vi "Gripper Controller.vi"(8 "error in":errorcluster) -> ()   [LabVIEW 2017]
doc: "This VI executes continuously carrying out the current operation and responding to updates or new operations. It will often contain the timing or control code that is difficult to place directly in TeleOp. This VI generally opens all sensors and motors and isolates the rest of the robot code from knowing how the operations are carried out."
uses:
  <vilib>/Rock Robotics/WPI/Framework/Completion Status.ctl
  Gripper Setpoints.ctl
  Gripper Operations.ctl
  <vilib>/Rock Robotics/SystemInterfaces/DIO/FPGA_DIOPWMChannel.ctl
  <vilib>/Rock Robotics/Network Tables/NT Write Boolean.vi
panel:
  in  "Interactive Values":T1
  out "Current\nCmd":string
  in  "Buttons":cluster{"Execute Cmd":bool, "Abort Cmd":bool}
  out "Command Timing":cluster{"Start Time (ms)":u32, "Iterations":i32}
  out "Status":T3
  # "Tip: It may be helpful to observe inputs and sensor values.\nYou may also want to display tuning or debugging controls."
  # "Interactive Command: You may fill in the settings for a command\nand schedule it with the Execute button. You can observe and abort\nany command while fine tuning the code for the controller."
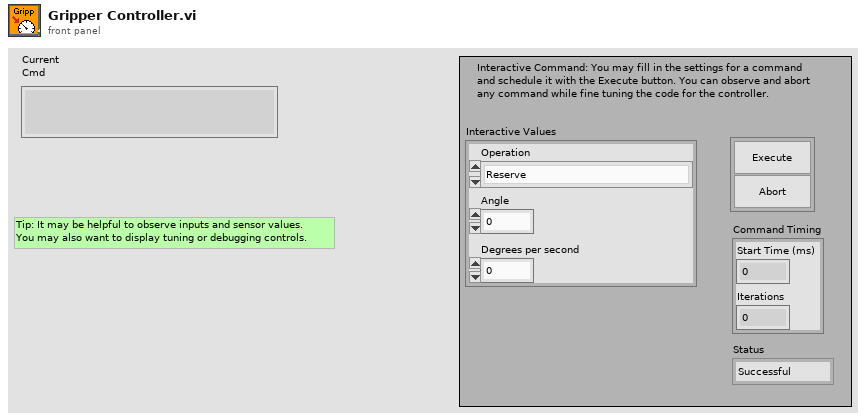
[diagram p1: front panel]
types:
  T1 = typedef "Gripper Setpoints.ctl" = cluster{"Operation":T2, "Angle":dbl, "Degrees per second":dbl}
  T2 = typedef "Gripper Operations.ctl" = enum16{"Reserve", "Read Current", "Immediate", "Grip Power Cube", "Release Power Cube"}
  T3 = typedef "Completion Status.ctl" = enum16{"Successful", "Aborted", "Incomplete"}
  T4 = typedef "FPGA_DIOPWMChannel.ctl" = enum8{"PWM 0", "PWM 1", "PWM 2", "PWM 3", "PWM 4", "PWM 5", "PWM 6", "PWM 7", "PWM 8", "PWM 9", "PWM MXP 0", "PWM MXP 1", "PWM MXP 2", "PWM MXP 3", "PWM MXP 4", "PWM MXP 5", "PWM MXP 6", "PWM MXP 7", "PWM MXP 8", "PWM MXP 9", "Invalid"}
  T5 = typedef "WPI_ServoDeviceRef.ctl" = cluster{"DeviceStatus":errorcluster, "PWM Channel":T4, "DeadBand":T6}
  T6 = typedef "WPI_PWMDeadband.ctl" = cluster{"Name":string, "maxPositivePwm":i32, "minPositivePwm":i32, "centerPwm":i32, "maxNegativePwm":i32, "minNegativePwm":i32, "angularRange":u16}
  T7 = typedef "Command Status Info.ctl" = cluster{"Name":string, "Status":T3, "notifier out":T8}
  T8 = typedef "Completion Notifier.ctl" = refnum<notifier>
  T9 = cluster{"Current Command":T1, "Command Timing":cluster{"Start Time (ms)":u32, "Iterations":i32}, "Command Arguments":cluster{"Command Info":T7, "Description":string, "Default Command":T1, "queue out":refnum<queue>, "Subsystem Name":string}}
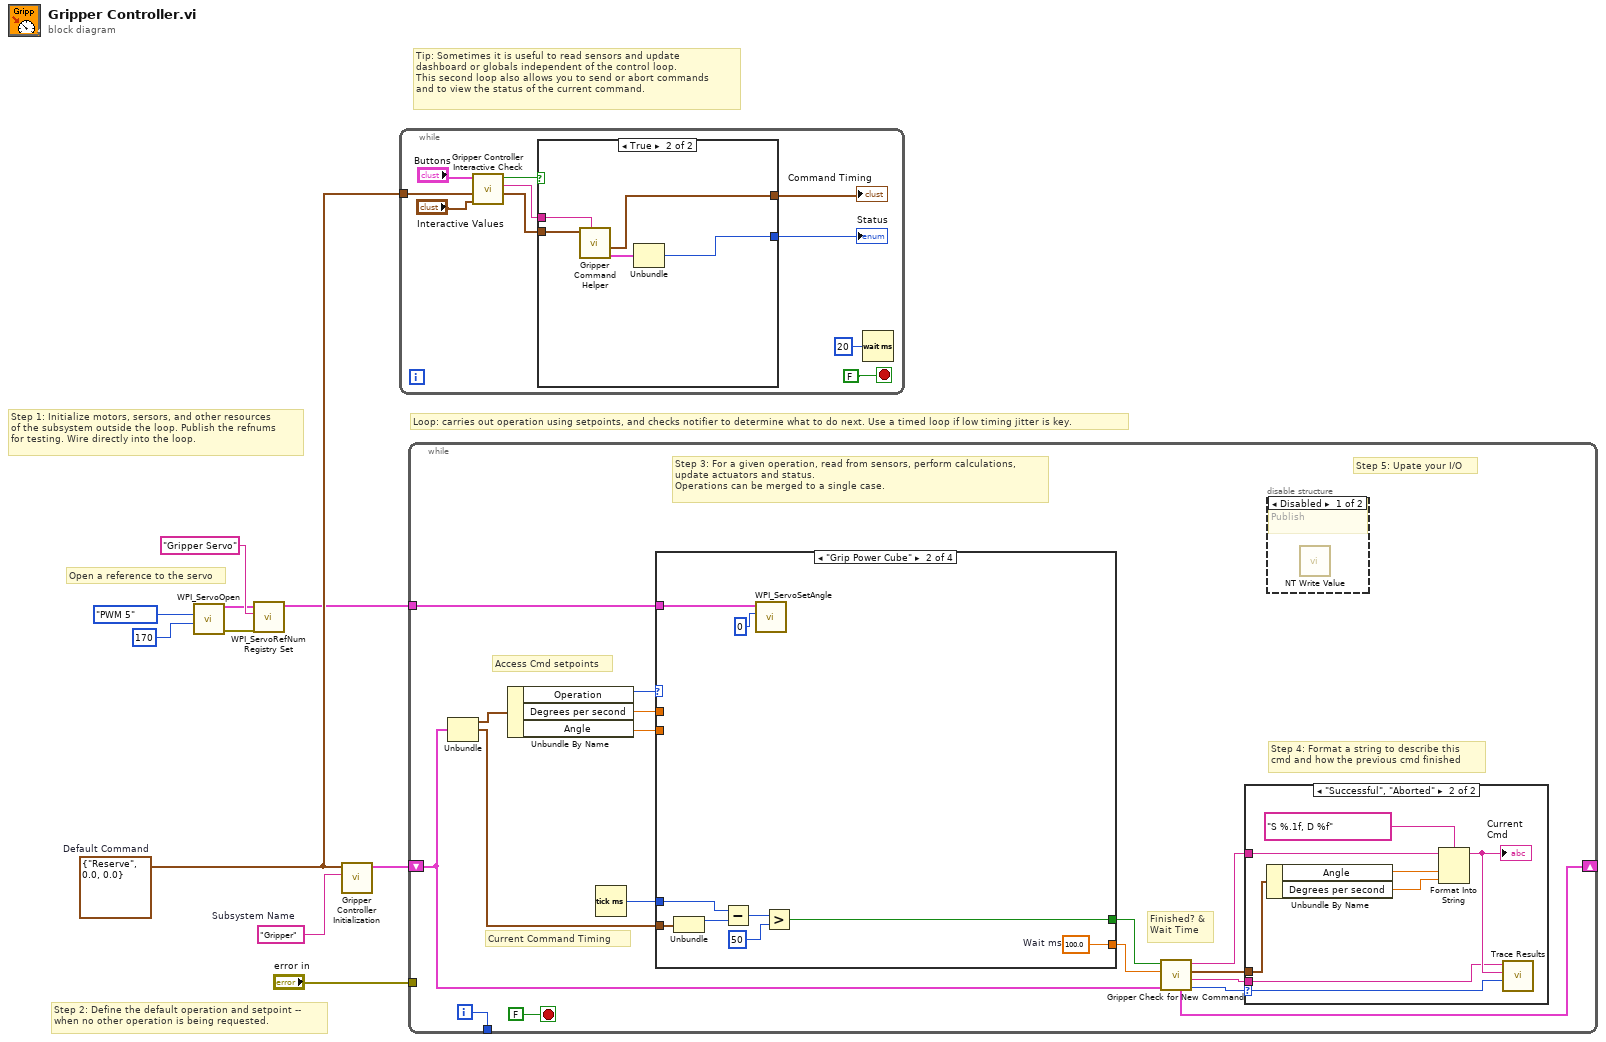
[diagram p0: block diagram]
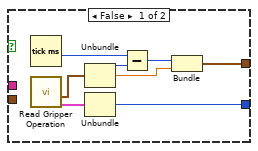
[diagram p2: hidden frame]
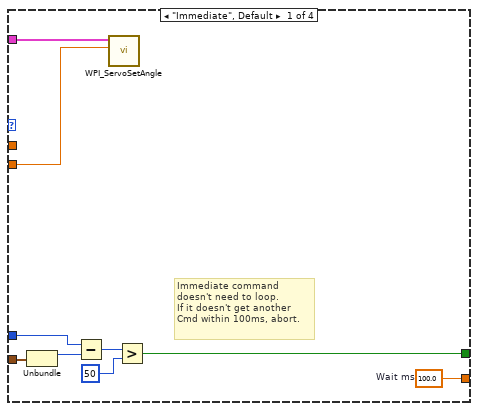
[diagram p5: hidden frame]
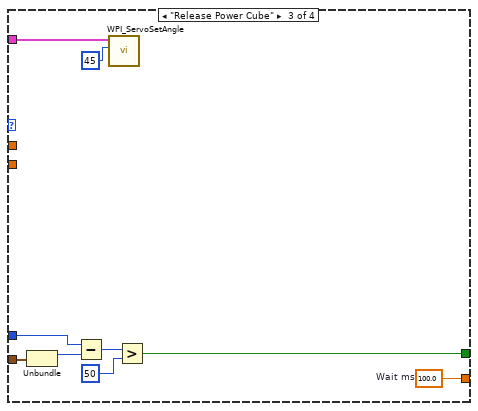
[diagram p6: hidden frame]
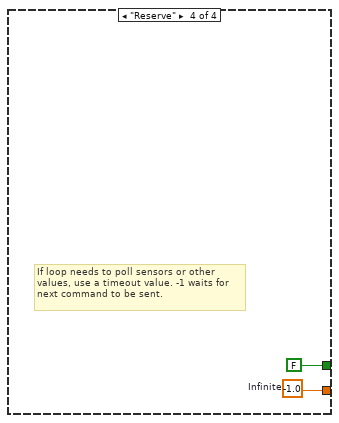
[diagram p7: hidden frame]
diagram:
  w7 = T1 {"Operation"=enum."Reserve", "Angle"=0.0, "Degrees per second"=0.0}  # Default Command
  w8 = "Gripper"  # Subsystem Name
  # "Open a reference to the servo"
  # "Tip: Sometimes it is useful to read sensors and update\ndashboard or globals independent of the control loop.\nThis second loop also allows you to send or abort commands\nand to view the status of the current command."
  # "Step 2: Define the default operation and setpoint --\nwhen no other operation is being requested."
  # "Step 1: Initialize motors, sersors, and other resources\nof the subsystem outside the loop. Publish the refnums\nfor testing. Wire directly into the loop."
  # "Loop: carries out operation using setpoints, and checks notifier to determine what to do next. Use a timed loop if low timing jitter is key."
  n1 = call <vilib>:"WPI_ServoOpen.vi"("Angular Range"=u16 170, "PWM Channel"=FPGA_DIOPWMChannel."PWM 5") -> ("error out"=w4:errorcluster, "ServoDeviceRef"=w5:T5)  [unwired: 2 in, 6 out]
  n2 = call <vilib>:"WPI_ServoRefNum Registry Set.vi"("error in (no error)"=w4, "refnum name"="Gripper Servo", "ServoDeviceRef"=w5) -> ("ServoDeviceRef"=w1:T5)  [unwired: 7 in, 1 out]
  n3 = call "Gripper Controller Initialization.vi"("Subsystem Name"=w8, "Default Command"=w7) -> ("Current Command"=w9:T9)  [unwired: 9 in]
  n4 = while {
    tunnel: w7 -> [w17]
    stop <- FALSE stop-if-true
    n5 = call "Gripper Controller Interactive Check.vi"("Interactive Command in"="Interactive Values", "Default Command"=w17, "Buttons"="Buttons") -> ("Interactive Command out"=w14:T1, "Trace String"=w15:string, "Schedule"=w16:bool)  [unwired: 6 in]
    n6 = case shown="True" w16 {
      tunnel: [w28 w33] -> w13
      tunnel: w14 -> [_ w31]
      tunnel: [w24 w29] -> w12
      tunnel: w15 -> [_ w32]
      frame False {
        n7 = Tick Count (ms)() -> (millisecond timer value=w23:u32)
        n8 = call "Read Gripper Operation.vi"() -> ("Command Info"=w21:T7, "SubSystem Data"=w22:T1)  [unwired: 9 in, 1 out]
        n9 = Unbundle(w22) -> ("Operation"=w27:T2, "Angle"=w25:dbl)  [unwired: 1 out]
        n10 = Unbundle(w21) -> ("Status"=w28:T3)  [unwired: 2 out]
        n11 = Subtract(x=w23, y=w27) -> (x-y=w26:u32)
        n12 = Bundle(w26, "Angle"=w25) -> (w24:cluster{u32, "Angle":dbl})  [unwired: 1 in]
      }
      frame True {
        n13 = call "Gripper Command Helper.vi"("Description"=w32, "SubSystem Data"=w31) -> ("Command Info Out"=w30:T7, "Command Timing"=w29:cluster{"Start Time (ms)":u32, "Iterations":i32})  [unwired: 7 in, 1 out]
        n14 = Unbundle(w30) -> ("Status"=w33:T3)  [unwired: 2 out]
      }
    }
    "Status" <- w13
    "Command Timing" <- w12
    n15 = Wait (ms)(milliseconds to wait=u32 20) -> ()  [unwired: 1 out]
  }
  n16 = while {
    shift-right: [w42] -> _
    shift-left: w9 -> [w35]
    tunnel: [w49] -> _
    tunnel: "error in" -> [_]
    tunnel: w1 -> [w34]
    i -> [w49]
    stop <- FALSE stop-if-true
    # "Step 5: Upate your I/O"
    # "Step 4: Format a string to describe this\ncmd and how the previous cmd finished"
    # "Current Command Timing"
    # "Access Cmd setpoints"
    # "Finished? &\nWait Time"
    # "Step 3: For a given operation, read from sensors, perform calculations,\nupdate actuators and status.\nOperations can be merged to a single case."
    n17 = Unbundle(w35) -> ("Current Command"=w48:T1, "Command Timing"=w44:cluster{"Start Time (ms)":u32, "Iterations":i32})  [unwired: 1 out]
    n18 = Unbundle By Name(w48) -> ("Operation"=w47:T2, "Degrees per second"=w46:dbl, "Angle"=w43:dbl)
    n19 = Tick Count (ms)() -> (millisecond timer value=w45:u32)
    n20 = case shown="\"Grip Power Cube\"" w47 {
      tunnel: [w67 w76 w85 w87] -> w40
      tunnel: [w61 w70 w79 FALSE ("ignore previous (F)")] -> w41
      tunnel: w44 -> [w63 w72 w81 _]
      tunnel: w46 -> [_ _ _ _]
      tunnel: w45 -> [w62 w71 w80 _]
      tunnel: w43 -> [w59 _ _ _]
      tunnel: w34 -> [w60 w68 w77 _]
      frame "Immediate", Default {
        w67 = 100.0  # Wait ms
        # "Immediate command\ndoesn't need to loop.\nIf it doesn't get another\nCmd within 100ms, abort."
        n21 = Unbundle(w63) -> ("Start Time (ms)"=w66:u32)  [unwired: 1 out]
        n22 = Subtract(x=w62, y=w66) -> (x-y=w65:u32)
        n23 = call <vilib>:"WPI_ServoSetAngle.vi"("Angle"=w59, "ServoDeviceRef"=w60) -> ()  [unwired: 8 in, 2 out]
        n24 = Greater?(x=w65, y=u8 50 ("Left Motor")) -> (0:w61:bool)
      }
      frame "Grip Power Cube" {
        w76 = 100.0  # Wait ms
        n25 = Unbundle(w72) -> ("Start Time (ms)"=w75:u32)  [unwired: 1 out]
        n26 = Subtract(x=w71, y=w75) -> (x-y=w74:u32)
        n27 = call <vilib>:"WPI_ServoSetAngle.vi"("Angle"=0, "ServoDeviceRef"=w68) -> ()  [unwired: 8 in, 2 out]
        n28 = Greater?(x=w74, y=u8 50 ("Left Motor")) -> (0:w70:bool)
      }
      frame "Release Power Cube" {
        w85 = 100.0  # Wait ms
        n29 = Unbundle(w81) -> ("Start Time (ms)"=w84:u32)  [unwired: 1 out]
        n30 = Subtract(x=w80, y=w84) -> (x-y=w83:u32)
        n31 = call <vilib>:"WPI_ServoSetAngle.vi"("Angle"=45, "ServoDeviceRef"=w77) -> ()  [unwired: 8 in, 2 out]
        n32 = Greater?(x=w83, y=u8 50 ("Left Motor")) -> (0:w79:bool)
      }
      frame "Reserve" {
        w87 = -1.0  # Infinite
        # "If loop needs to poll sensors or other\nvalues, use a timeout value. -1 waits for\nnext command to be sent."
      }
    }
    n33 = call "Gripper Check for New Command.vi"("Current Command"=w35, "Wait time (ms)"=w40, "Finished?"=w41) -> ("Completion"=w36:T3, "Subsystem Name"=w37:string, "Current Command"=w38:T1, "Initial Trace String"=w39:string, "NextCommand"=w42:T9)  [unwired: 4 in]
    n34 = case shown="\"Successful\", \"Aborted\"" w36 {
      selector: w36 -> [_ w58]
      tunnel: w39 -> [_ w54]
      tunnel: w38 -> [_ w55]
      tunnel: w37 -> [_ w51]
      frame "Incomplete", Default {
        # "Continuing current command"
      }
      frame "Successful", "Aborted" {
        # "Report and setup for next command"
        n35 = Unbundle By Name(w55) -> ("Angle"=w57:dbl, "Degrees per second"=w52:dbl)
        n36 = Format Into String(format string="S %.1f, D %f", initial string=w54, w57, w52) -> (resulting string=w53:string)  [unwired: 1 in, 1 out]
        "Current\nCmd" <- w53
        n37 = call <vilib>:"Trace Results.vi"("Status of previous command"=w58, "Description"=w53, "Subsystem"=w51) -> ()  [unwired: 9 in]
      }
    }
    n38 = disable-structure shown="Disabled" {
      frame Disabled {
        # "Publish"
        n39 = call-poly <vilib>:"NT Write Value.vi"() -> ()  [unwired: 11 in, 1 out]
      }
      frame Enabled {
      }
    }
  }
